vi "Motors Sub 01.vi"(7 "Cluster":T1, 8 "Error In":errorcluster, 11 "VISA in":refnum<visa-resource-name>) -> (0 "error out":errorcluster, 3 "VISA out":refnum<visa-resource-name>)   [LabVIEW 2010]
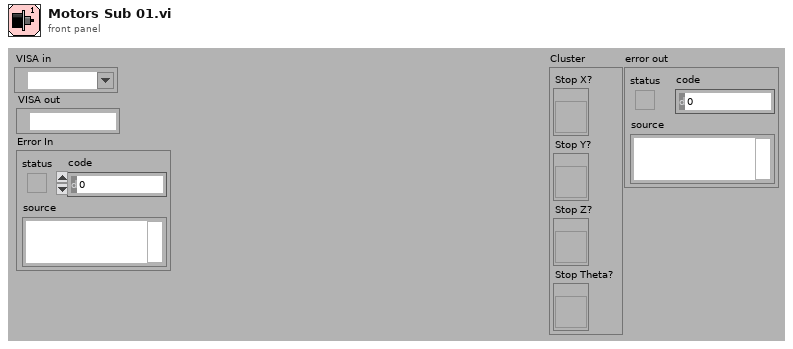
[diagram p1: front panel]
types:
  T1 = cluster{"Stop X?":refnum<vi>, "Stop Y?":refnum<vi>, "Stop Z?":refnum<vi>, "Stop Theta?":refnum<vi>}
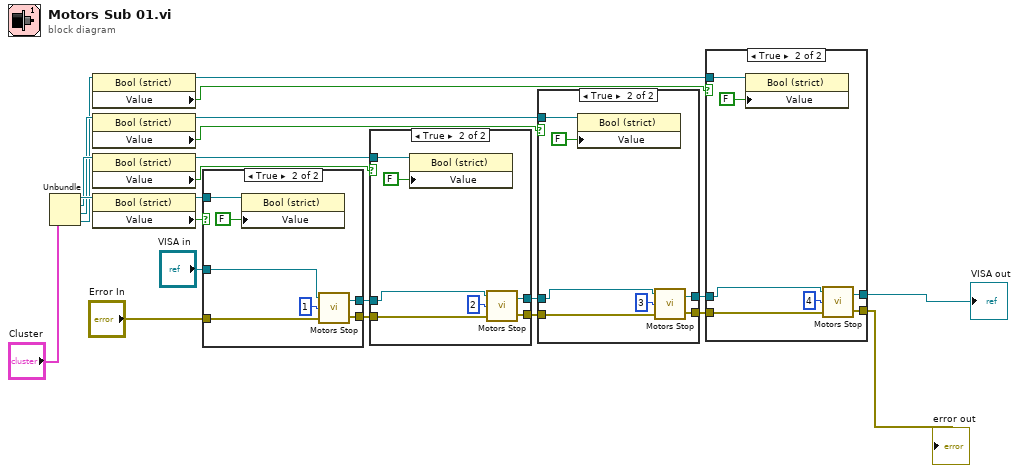
[diagram p0: block diagram]
diagram:
  n1 = Unbundle("Cluster") -> ("Stop X?"=w7:refnum<vi>, "Stop Y?"=w6:refnum<vi>, "Stop Z?"=w5:refnum<vi>, "Stop Theta?"=w4:refnum<vi>)
  n2 = property on="Property Node" class="Bool (strict)"(reference=w4) -> (reference out=w13:refnum<vi>, "Value"=w14:bool)  [unwired: 1 in, 1 out]
  n3 = property on="Property Node" class="Bool (strict)"(reference=w5) -> (reference out=w12:refnum<vi>, "Value"=w15:bool)  [unwired: 1 in, 1 out]
  n4 = property on="Property Node" class="Bool (strict)"(reference=w6) -> (reference out=w11:refnum<vi>, "Value"=w16:bool)  [unwired: 1 in, 1 out]
  n5 = property on="Property Node" class="Bool (strict)"(reference=w7) -> (reference out=w10:refnum<vi>, "Value"=w17:bool)  [unwired: 1 in, 1 out]
  n6 = case shown="True" w17 {
    tunnel: "Error In" -> [w24 w32]
    tunnel: "VISA in" -> [w25 w31]
    tunnel: [w25 w29] -> w18
    tunnel: [w24 w28] -> w19
    tunnel: w10 -> [_ w26]
    frame False {
    }
    frame True {
      n7 = property on="Property Node" class="Bool (strict)"(reference=w26, "Value"=FALSE) -> ()  [unwired: 1 in, 2 out]
      n8 = call "Motors Stop.vi"("error in"=w32, "Axis"=1, "VISA in"=w31) -> ("error out"=w28:errorcluster, "VISA out"=w29:refnum<visa-resource-name>)
    }
  }
  n9 = case shown="True" w16 {
    tunnel: w19 -> [w33 w41]
    tunnel: w18 -> [w34 w40]
    tunnel: [w34 w38] -> w20
    tunnel: [w33 w37] -> w21
    tunnel: w11 -> [_ w35]
    frame False {
    }
    frame True {
      n10 = property on="Property Node" class="Bool (strict)"(reference=w35, "Value"=FALSE) -> ()  [unwired: 1 in, 2 out]
      n11 = call "Motors Stop.vi"("error in"=w41, "Axis"=2, "VISA in"=w40) -> ("error out"=w37:errorcluster, "VISA out"=w38:refnum<visa-resource-name>)
    }
  }
  n12 = case shown="True" w15 {
    tunnel: w21 -> [w42 w50]
    tunnel: w20 -> [w43 w49]
    tunnel: [w43 w47] -> w22
    tunnel: [w42 w46] -> w23
    tunnel: w12 -> [_ w44]
    frame False {
    }
    frame True {
      n13 = property on="Property Node" class="Bool (strict)"(reference=w44, "Value"=FALSE) -> ()  [unwired: 1 in, 2 out]
      n14 = call "Motors Stop.vi"("error in"=w50, "Axis"=3, "VISA in"=w49) -> ("error out"=w46:errorcluster, "VISA out"=w47:refnum<visa-resource-name>)
    }
  }
  n15 = case shown="True" w14 {
    tunnel: w23 -> [w51 w59]
    tunnel: w22 -> [w52 w58]
    tunnel: [w52 w56] -> w8
    tunnel: [w51 w55] -> w3
    tunnel: w13 -> [_ w53]
    frame False {
    }
    frame True {
      n16 = property on="Property Node" class="Bool (strict)"(reference=w53, "Value"=FALSE) -> ()  [unwired: 1 in, 2 out]
      n17 = call "Motors Stop.vi"("error in"=w59, "Axis"=4, "VISA in"=w58) -> ("error out"=w55:errorcluster, "VISA out"=w56:refnum<visa-resource-name>)
    }
  }
  "VISA out" <- w8
  "error out" <- w3
